vi "Instr_SetPrivateData.vi"(8 "error in (no error)":errorcluster, 11 "KE2410 in":refnum<class "KE2410.lvclass">) -> (0 "error out":errorcluster, 3 "KE2410 out":refnum<class "KE2410.lvclass">)   [LabVIEW 2013, in "KE2410.lvclass"]
uses:
  KE2410.lvclass
  KE2410_CommandsGlobal.vi
  InstrumentSetup.vi
  InstrControl.lvclass
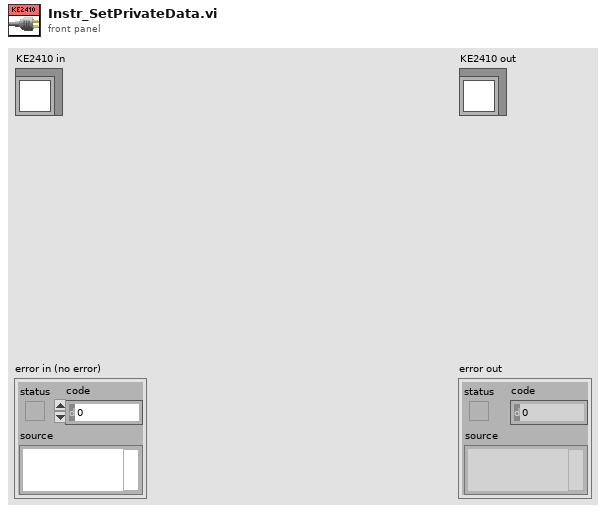
[diagram p1: front panel]
types:
  T1 = cluster{"Current Limit":sgl, "GPIB Address":string}
  T2 = cluster{"GPIB address":string, "Instrument name":string, "Instrument type":u16, "Command \"Reset\"":string, "Command \"Initialise\"":string, "Command \"Arm\"":string, "Command \"SetVolts\"":string, "Command \"Compliance?\"":string, "Command \"Standby\"":string, "Command \"Read Current\"":string}
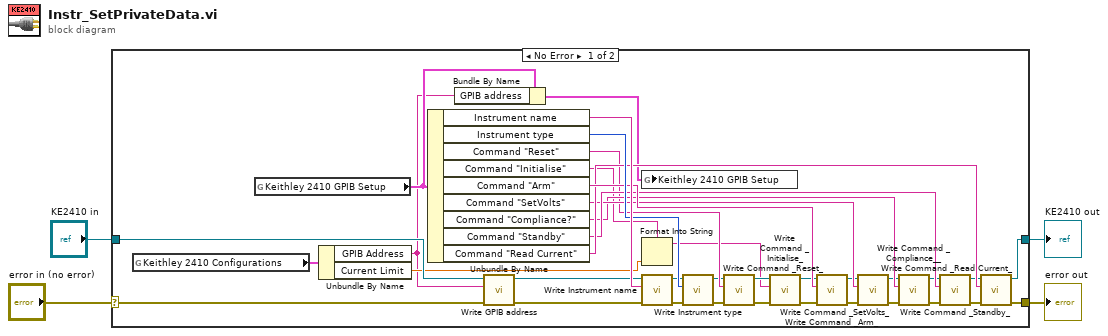
[diagram p0: block diagram]
diagram:
  n1 = case shown="No Error" "error in (no error)" {
    selector: "error in (no error)" -> [w24 w43]
    tunnel: [w13 w43] -> w3
    tunnel: [w14 w42] -> w1
    tunnel: "KE2410 in" -> [w12 w42]
    frame No Error {
      n2 = global read "InstrumentSetup.vi" "Keithley 2410 Configurations"() -> (w11:T1)
      n3 = global read "KE2410_CommandsGlobal.vi" "Keithley 2410 GPIB Setup"() -> (w6:T2)
      n4 = Unbundle By Name(w11) -> ("GPIB Address"=w5:string, "Current Limit"=w10:sgl)
      n5 = Unbundle By Name(w6) -> ("Instrument name"=w41:string, "Instrument type"=w40:u16, "Command \"Reset\""=w34:string, "Command \"Initialise\""=w9:string, "Command \"Arm\""=w39:string, "Command \"SetVolts\""=w36:string, "Command \"Compliance?\""=w35:string, "Command \"Standby\""=w37:string, "Command \"Read Current\""=w38:string)
      n6 = Bundle By Name(cluster=w6, "GPIB address"=w5) -> (w7:T2)
      n7 = call-dynamic "Write GPIB address.vi"("error in (no error)"=w24, "GPIB address"=w5, "InstControl in"=w12) -> ("error out"=w23:errorcluster, "InstControl out"=w33:refnum<class "KE2410.lvclass">)  [unwired: 7 in]
      n8 = global write "KE2410_CommandsGlobal.vi" "Keithley 2410 GPIB Setup"(w7) -> ()
      n9 = Format Into String(format string=w9, w10) -> (resulting string=w8:string)  [unwired: 2 in, 1 out]
      n10 = call-dynamic "Write Instrument name.vi"("error in (no error)"=w23, "Instrument name"=w41, "InstControl in"=w33) -> ("error out"=w22:errorcluster, "InstControl out"=w32:refnum<class "KE2410.lvclass">)  [unwired: 7 in]
      n11 = call-dynamic "Write Instrument type.vi"("error in (no error)"=w22, "Instrument type"=w40, "InstControl in"=w32) -> ("error out"=w21:errorcluster, "InstControl out"=w31:refnum<class "KE2410.lvclass">)  [unwired: 7 in]
      n12 = call-dynamic "Write Command _Reset_.vi"("error in (no error)"=w21, "Command \"Reset\""=w34, "SupplyControl in"=w31) -> ("error out"=w20:errorcluster, "SupplyControl out"=w30:refnum<class "KE2410.lvclass">)  [unwired: 7 in]
      n13 = call-dynamic "Write Command _Initialise_.vi"("error in (no error)"=w20, "Command \"Initialise\""=w8, "SupplyControl in"=w30) -> ("error out"=w19:errorcluster, "SupplyControl out"=w29:refnum<class "KE2410.lvclass">)  [unwired: 7 in]
      n14 = call-dynamic "Write Command _Arm_.vi"("error in (no error)"=w19, "Command \"Arm\""=w39, "SupplyControl in"=w29) -> ("error out"=w18:errorcluster, "SupplyControl out"=w28:refnum<class "KE2410.lvclass">)  [unwired: 7 in]
      n15 = call-dynamic "Write Command _SetVolts_.vi"("error in (no error)"=w18, "Command \"SetVolts\""=w36, "SupplyControl in"=w28) -> ("error out"=w17:errorcluster, "SupplyControl out"=w27:refnum<class "KE2410.lvclass">)  [unwired: 7 in]
      n16 = call-dynamic "Write Command _Compliance__.vi"("error in (no error)"=w17, "Command \"Compliance?\""=w35, "SupplyControl in"=w27) -> ("error out"=w16:errorcluster, "SupplyControl out"=w26:refnum<class "KE2410.lvclass">)  [unwired: 7 in]
      n17 = call-dynamic "Write Command _Standby_.vi"("error in (no error)"=w16, "Command \"Standby\""=w37, "SupplyControl in"=w26) -> ("error out"=w15:errorcluster, "SupplyControl out"=w25:refnum<class "KE2410.lvclass">)  [unwired: 7 in]
      n18 = call-dynamic "Write Command _Read Current_.vi"("error in (no error)"=w15, "Command \"Read Current\""=w38, "SupplyControl in"=w25) -> ("error out"=w13:errorcluster, "SupplyControl out"=w14:refnum<class "KE2410.lvclass">)  [unwired: 7 in]
    }
    frame Error {
    }
  }
  "error out" <- w3
  "KE2410 out" <- w1
